vi "test Compare Ports Between Import and Sysdef.vi"(8 "error in":errorcluster, 11 "TestCase in":refnum<class "Refresh.lvclass">) -> (0 "error out":errorcluster, 3 "TestCase out":refnum<class "Refresh.lvclass">)   [LabVIEW 2020, in "Refresh.lvclass"]
uses:
  Refresh.lvclass
  <vilib>/addons/_JKI Toolkits/VI Tester/TestCase.llb/TestCase.lvclass
  <vilib>/NI/VeriStand Custom Device Testing Tools/VeriStandTestUtilities/VeriStandTestUtilities.lvlib
  Scripting/Ballard/Ballard ARINC 429 Scripting.lvlib
  Import/ARINC 429 Import.lvlib
  System Explorer/Implementation/Implementation.lvlib
  C:/Program Files (x86)/National Instruments/LabVIEW 2020/vi.lib/addons/_JKI Toolkits/VI Tester/TestCase.llb/TestCase.lvclass
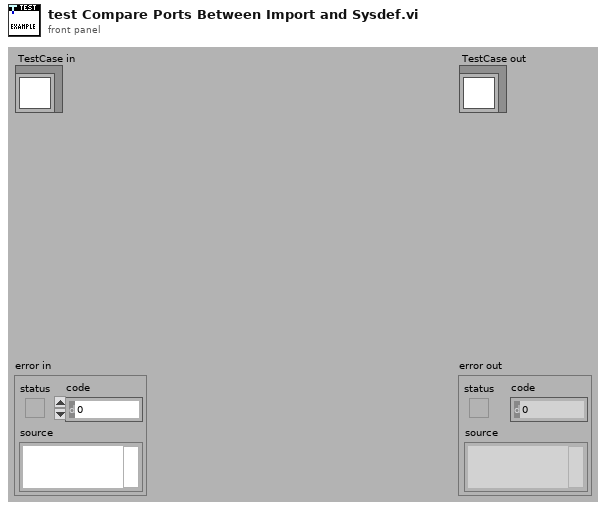
[diagram p1: front panel]
types:
  T1 = typedef "VS Channels Definition for All Labels on Hardware Channel.ctl" = cluster{"hardware channel":i32, "direction":T2, "labels":T3[], "speed":T8}
  T2 = typedef "Direction.ctl" = enum16{"Rx", "Tx"}
  T3 = typedef "VS Channels Definition for Label.ctl" = cluster{"label (Dec)":u32, "parameters":T4[], "SDI value":u8, "SDI enabled":bool, "transfer type":T7, "create timestamp":bool, "transmit period":u32}
  T4 = typedef "VS Channel Definition for Parameter.ctl" = cluster{"name":string, "default value":dbl, "unit":string, "Parameter":T5}
  T5 = typedef "Parameter Definition.ctl" = cluster{"start index":i32, "size":i32, "encoding":T6, "signed":bool, "scale multiplier":dbl, "scale offset":dbl}
  T6 = typedef "Encoding and Decoding.lvlib/Encoding.ctl" = enum16{"BNR", "BCD", "Discrete"}
  T7 = typedef "Transfer Type.ctl" = enum16{"Scheduled", "Acyclic", "Block", "Strobe"}
  T8 = typedef "Transfer Speed.ctl" = enum16{"LO (12.5 kb/s)", "HI (100 kb/s)"}
  T9 = typedef "Custom Device API.lvlib/Custom Device Item Ref.ctl" = u64
  T10 = typedef "Ballard ARINC 429 System Explorer.lvlib/Implementation.lvlib/Refresh Listbox.ctl" = cluster{"Item Names":string[], "Item Symbol":T11, "Change Flag":bool}
  T11 = typedef "Ballard ARINC 429 System Explorer.lvlib/Implementation.lvlib/Refresh Symbols.ctl" = enum16{"Blank", "Port", "Incoming", "Outgoing", "Label", "Word", "Parameter", "ARINC-429", "Config Files", "Channel Spec", "Item"}
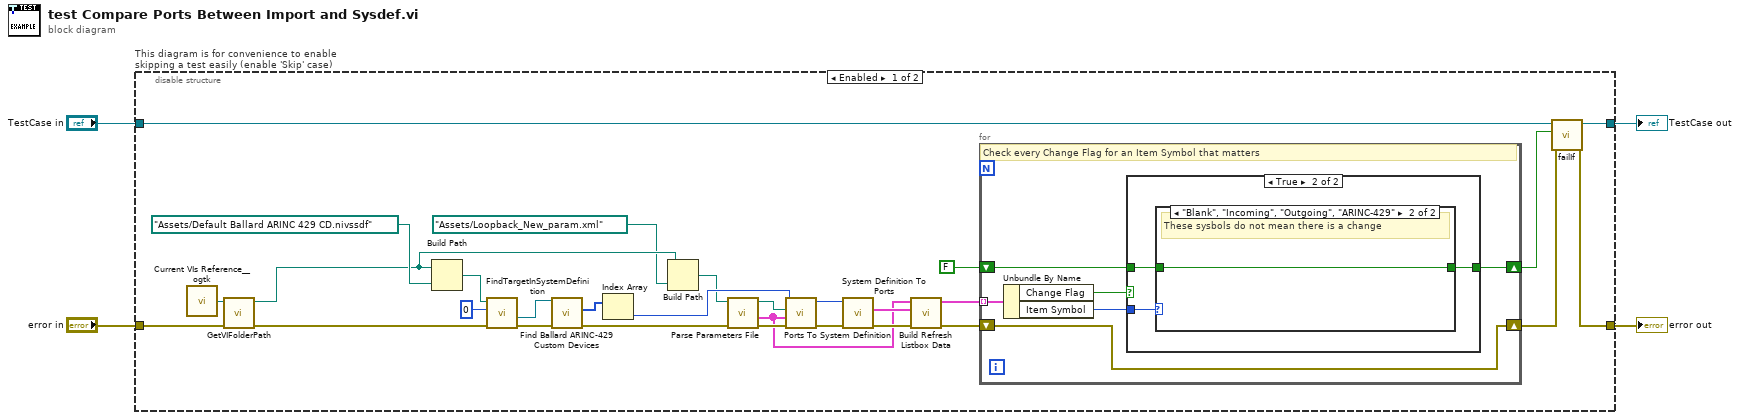
[diagram p0: block diagram]
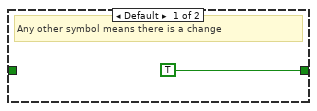
[diagram p3: hidden frame]
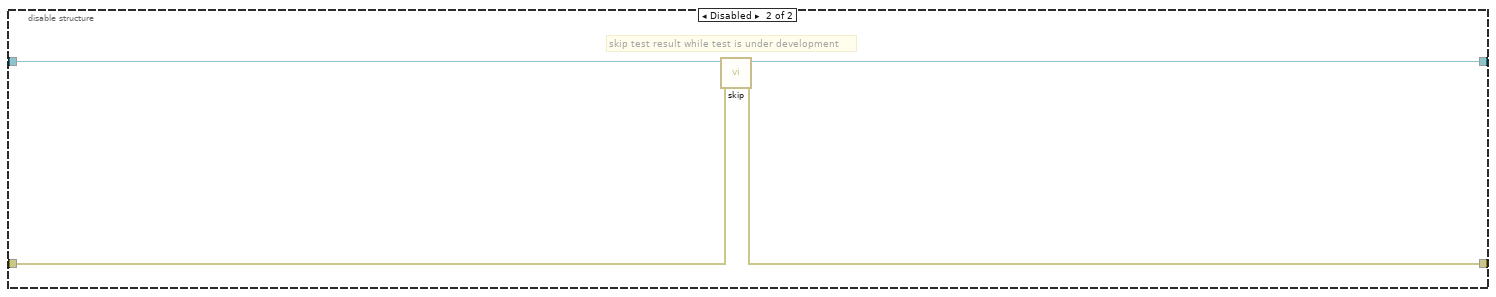
[diagram p4: hidden frame]
diagram:
  n1 = disable-structure "This diagram is for convenience to enable skipping a test easily (enable 'Skip' case)" shown="Enabled" {
    disable-tunnel: "TestCase in" -> [w5 w48]
    disable-tunnel: [w10 w49] -> w1
    disable-tunnel: [w6 w46] -> w3
    disable-tunnel: "error in" -> [w29 w47]
    frame Enabled {
      n2 = call <userlib>:"Current VIs Reference__ogtk.vi"() -> ("Current VI's reference"=w30:refnum<vi>)  [unwired: 5 in]
      n3 = call <vilib>:"GetVIFolderPath.vi"("error in (no error)"=w29, "VI Reference in"=w30) -> ("error out"=w33:errorcluster, "VI Folder Path out"=w24:path)  [unwired: 8 in]
      n4 = Build Path(base path=w24, name or relative path=path "Assets/Default Ballard ARINC 429 CD.nivssdf" ("Absolute or Relative Path")) -> (appended path=w31:path)
      n5 = call <vilib>:"FindTargetInSystemDefinition.vi"("error in"=w33, "target index"=0 ("index"), "system definition path"=w31) -> ("error out"=w27:errorcluster, "Target"=w26:refnum<k24>)  [unwired: 5 in, 2 out]
      n6 = call "Find Ballard ARINC-429 Custom Devices.vi"("error in"=w27, "target in"=w26) -> ("error out"=w18:errorcluster, "Ballard ARINC 429 custom devices"=w28:u64[])  [unwired: 7 in, 1 out]
      n7 = Index Array(array=w28) -> (element=w20:u64)  [unwired: 1 in]
      n8 = Build Path(base path=w24, name or relative path=path "Assets/Loopback_New_param.xml" ("Absolute or Relative Path")) -> (appended path=w19:path)
      n9 = call "Parse Parameters File.vi"("error in"=w18, "path to XML document"=w19) -> ("error out"=w21:errorcluster, "ports"=w13:T1[], "path to XML document out"=w22:path)  [unwired: 7 in]
      n10 = call "Ports To System Definition.vi"("error in"=w21, "ports"=w13, "parameter configuration file path"=w22, "custom device ref"=w20) -> ("error out"=w16:errorcluster, "custom device ref out"=w17:T9)  [unwired: 6 in]
      n11 = call "System Definition To Ports.vi"("error in"=w16, "custom device ref"=w17) -> ("error out"=w15:errorcluster, "ports"=w14:T1[])  [unwired: 7 in, 1 out]
      n12 = call "Build Refresh Listbox Data.vi"("error in"=w15, "new ports"=w14, "current ports"=w13) -> ("error out"=w8:errorcluster, "refresh listbox"=w12:T10[])  [unwired: 7 in]
      n13 = for {
        tunnel: w12 -> [w39] mode=indexing
        shift-right: [w35] -> w9
        shift-left: FALSE -> [w36]
        shift-right: [w34] -> w7
        shift-left: w8 -> [w34]
        # "Check every Change Flag for an Item Symbol that matters"
        n14 = Unbundle By Name(w39) -> ("Change Flag"=w38:bool, "Item Symbol"=w37:T11)
        n15 = case shown="True" w38 {
          tunnel: w37 -> [_ w43]
          tunnel: w36 -> [w40 w42]
          tunnel: [w40 w41] -> w35
          frame False {
          }
          frame True {
            n16 = case shown="\"Blank\", \"Incoming\", \"Outgoing\", \"ARINC-429\"" w43 {
              tunnel: w42 -> [_ w45]
              tunnel: [TRUE w45] -> w41
              frame Default {
                # "Any other symbol means there is a change"
              }
              frame "Blank", "Incoming", "Outgoing", "ARINC-429" {
                # "These sysbols do not mean there is a change"
              }
            }
          }
        }
      }
      n17 = call-dynamic "failIf.vi"("error in (no error)"=w7, "fail"=w9, "TestCase in"=w5) -> ("error out"=w6:errorcluster, "TestCase out"=w10:refnum<class "Refresh.lvclass">)  [unwired: 7 in]
    }
    frame Disabled {
      # "skip test result while test is under development"
      n18 = call <vilib>:"skip.vi"("error in (no error)"=w47, "TestCase in"=w48) -> ("error out"=w46:errorcluster, "TestCase out"=w49:refnum<class "Refresh.lvclass">)  [unwired: 8 in]
    }
  }
  "error out" <- w3
  "TestCase out" <- w1
